vi "Read Key.vi"(8 "Error In":errorcluster, 11 "Keyable In":refnum<class "Keyable.lvclass">) -> (0 "Error Out":errorcluster, 2 "Key":string, 3 "Keyable Out":refnum<class "Keyable.lvclass">)   [LabVIEW 2018, in "Toolkit.lvlib" / "Tokens.lvlib" / "Keyable.lvclass"]
doc: "Gets the key to the Mustache tag that uniquely identifies within the template. Any tag with the same key will be rendered with the same data.\n\n<B>Keyable In/Out</B> - A token that has a key, or name.\n\n<B>Key</B> - The name of the token."
uses:
  Keyable.lvclass
  Keyable.lvclass/Keyable.ctl
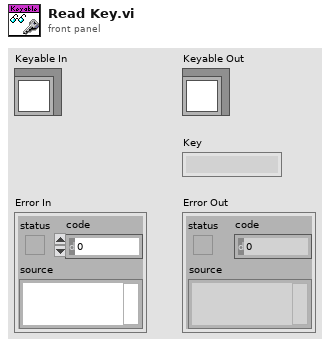
[diagram p1: front panel]
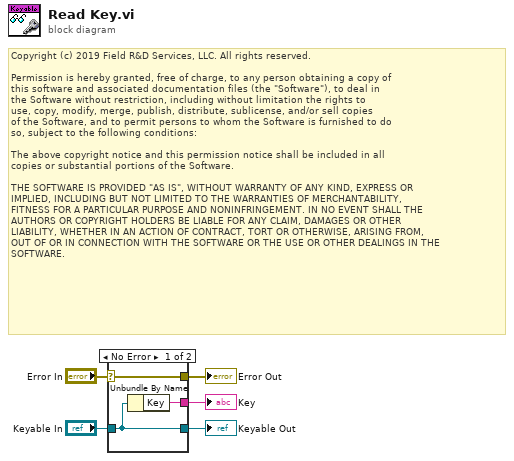
[diagram p0: block diagram]
diagram:
  # "Copyright (c) 2019 Field R&D Services, LLC. All rights reserved.\n\nPermission is hereby granted, free of charge, to any person obtaining a copy of\nthis software and associated documentation files (the \"Software\"), to deal in\nthe Software without restriction, including without limitation the rights to\nuse, copy, modify, merge, publish, distribute, sublicense, and/or sell copies\nof the Software, and to permit persons to whom the Software is furnished to do\nso, subject to the following conditions:\n\nThe above copyright notice and this permission notice shall be included in all\ncopies or substantial portions of the Software.\n\nTHE SOFTWARE IS PROVIDED \"AS IS\", WITHOUT WARRANTY OF ANY KIND, EXPRESS OR\nIMPLIED, INCLUDING BUT NOT LIMITED TO THE WARRANTIES OF MERCHANTABILITY,\nFITNESS FOR A PARTICULAR PURPOSE AND NONINFRINGEMENT. IN NO EVENT SHALL THE\nAUTHORS OR COPYRIGHT HOLDERS BE LIABLE FOR ANY CLAIM, DAMAGES OR OTHER\nLIABILITY, WHETHER IN AN ACTION OF CONTRACT, TORT OR OTHERWISE, ARISING FROM,\nOUT OF OR IN CONNECTION WITH THE SOFTWARE OR THE USE OR OTHER DEALINGS IN THE\nSOFTWARE."
  n1 = case shown="No Error" "Error In" {
    selector: "Error In" -> [w8 w9]
    tunnel: [w8 w9] -> w4
    tunnel: "Keyable In" -> [w6 w10]
    tunnel: [w7 _] -> w2
    tunnel: [w6 w10] -> w1
    frame No Error {
      n2 = Unbundle By Name(w6) -> ("Key"=w7:string)
    }
    frame Error {
    }
  }
  "Error Out" <- w4
  "Keyable Out" <- w1
  "Key" <- w2
